vi "Read address.vi"(9 "Downloader in":refnum<class "Downloader.lvclass">) -> (3 "Downloader out":refnum<class "Downloader.lvclass">, 4 "address":string="192.168.1.7")   [LabVIEW 2014, in "Downloader.lvclass"]
uses:
  Downloader.lvclass
  Downloader.lvclass/Downloader.ctl
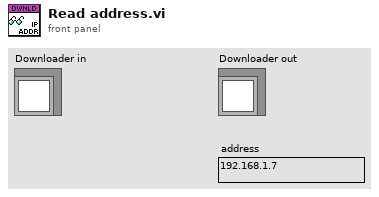
[diagram p1: front panel]
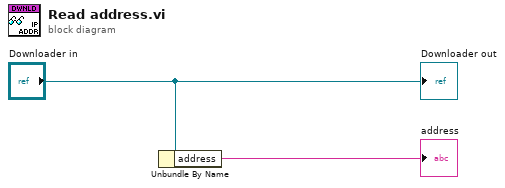
[diagram p0: block diagram]
diagram:
  n1 = Unbundle By Name("Downloader in") -> ("address"=→"address":string)
  "Downloader out" <- "Downloader in"
